vi "slopes2phase.vi"(5 "TypePhase":T1=enum."Modal_Zernike", 7 "Number of coefficients":u8=32, 8 "error in (no error)":errorcluster, 9 "Filter":u8[](array[numeric]), 10 "HasoSlopes in":refnum<class "HasoSlopes.lvclass">, 11 "Phase in":refnum<class "Phase.lvclass">) -> (0 "error out":errorcluster, 2 "HasoSlopes out":refnum<class "HasoSlopes.lvclass">, 3 "Phase out":refnum<class "Phase.lvclass">)   [LabVIEW 2018]
uses:
  <userlib>/WaveKit.lib/Classes/Phase/Phase.lvclass
  <userlib>/WaveKit.lib/Controls/WavefrontReconstructionMode.ctl
  <userlib>/WaveKit.lib/Controls/HasoSlopes.lvclass
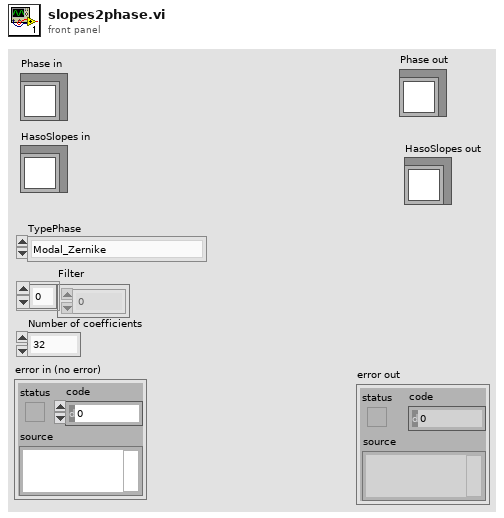
[diagram p1: front panel]
types:
  T1 = typedef "WavefrontReconstructionMode.ctl" = enum16{"None", "Modal_Legendre", "Modal_Zernike", "Zonal", "Modal_Zonal_Zernike", "Modal_Zonal_Legendre"}
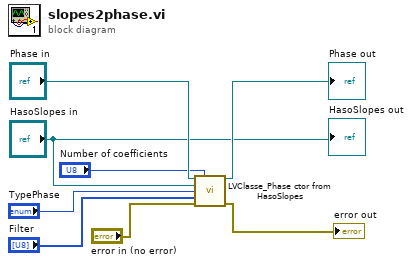
[diagram p0: block diagram]
diagram:
  n1 = call <userlib>:"LVClasse_Phase ctor from HasoSlopes.vi"("Phase in"="Phase in", "Number of coefficients"="Number of coefficients", "HasoSlopes.lvclass"="HasoSlopes in", "TypePhase"="TypePhase", "Filter"="Filter", "error in (no error)"="error in (no error)") -> ("Phase out"=→"Phase out":refnum<class "Phase.lvclass">, "error out"=→"error out":errorcluster)  [unwired: 8 in]
  "HasoSlopes out" <- "HasoSlopes in"
